vi "display_projector_one_color.vi"() -> ()   [LabVIEW 2019]
uses:
  <vilib>/vision/driver/IMAQdx.llb/IMAQdx Acquisition Mode.ctl
  ParametersGlobal.vi
  <vilib>/vision/NI_Vision_Development_Module.lvlib
  <vilib>/vision/driver/NI_Vision_Acquisition_Software.lvlib
panel:
  out "Processed Image":T1(plugin-control)
  out "Acquired Image 2":T1(plugin-control)
  out "Acquired Image":T1(plugin-control)
  in  "Single Color (T) Spatial Calibration Image (F)":bool=TRUE
  out "error out":errorcluster
  in  "Color Pixel Value":u32(colorbox)
  in  "Done":bool
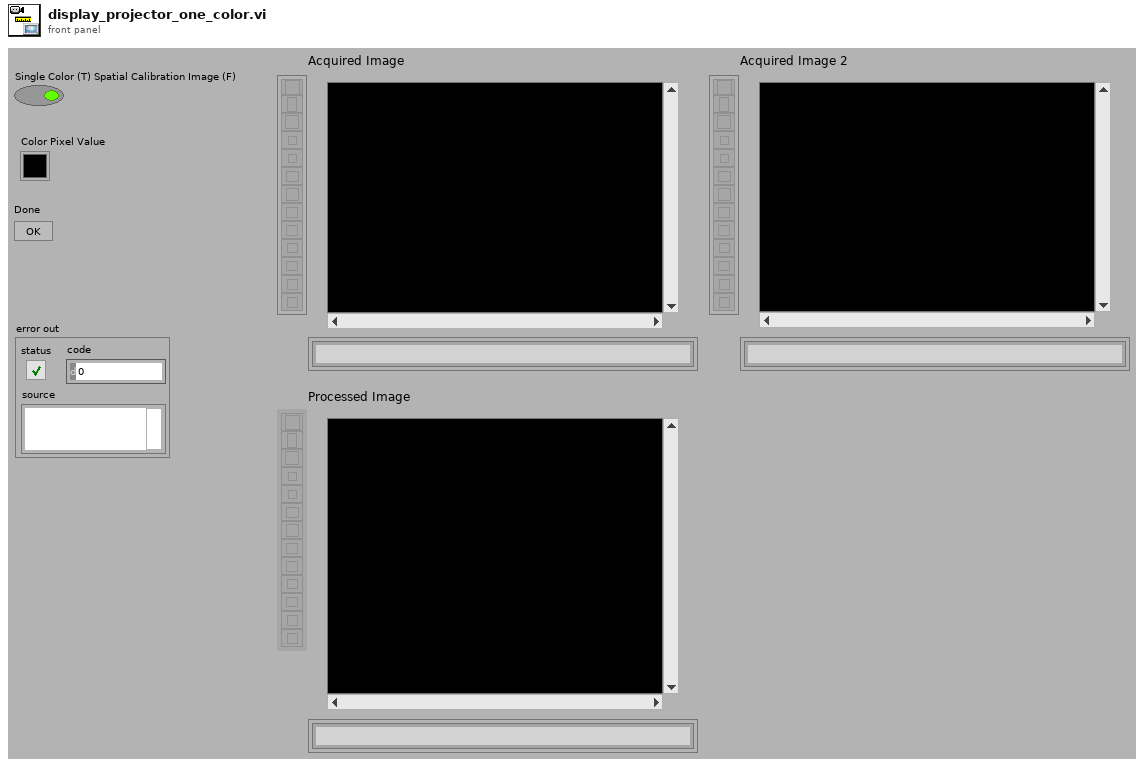
[diagram p1: front panel]
types:
  T1 = typedef "IMAQ Image.ctl" = refnum<image>
  T2 = typedef "NI_Vision_Acquisition_Software.lvlib/IMAQdx Acquisition Mode.ctl" = enum32{"One Shot", "Continuous"}
  T3 = typedef "Image Type" = u32
  T4 = typedef "IMAQdx.ctl" = refnum<k21>
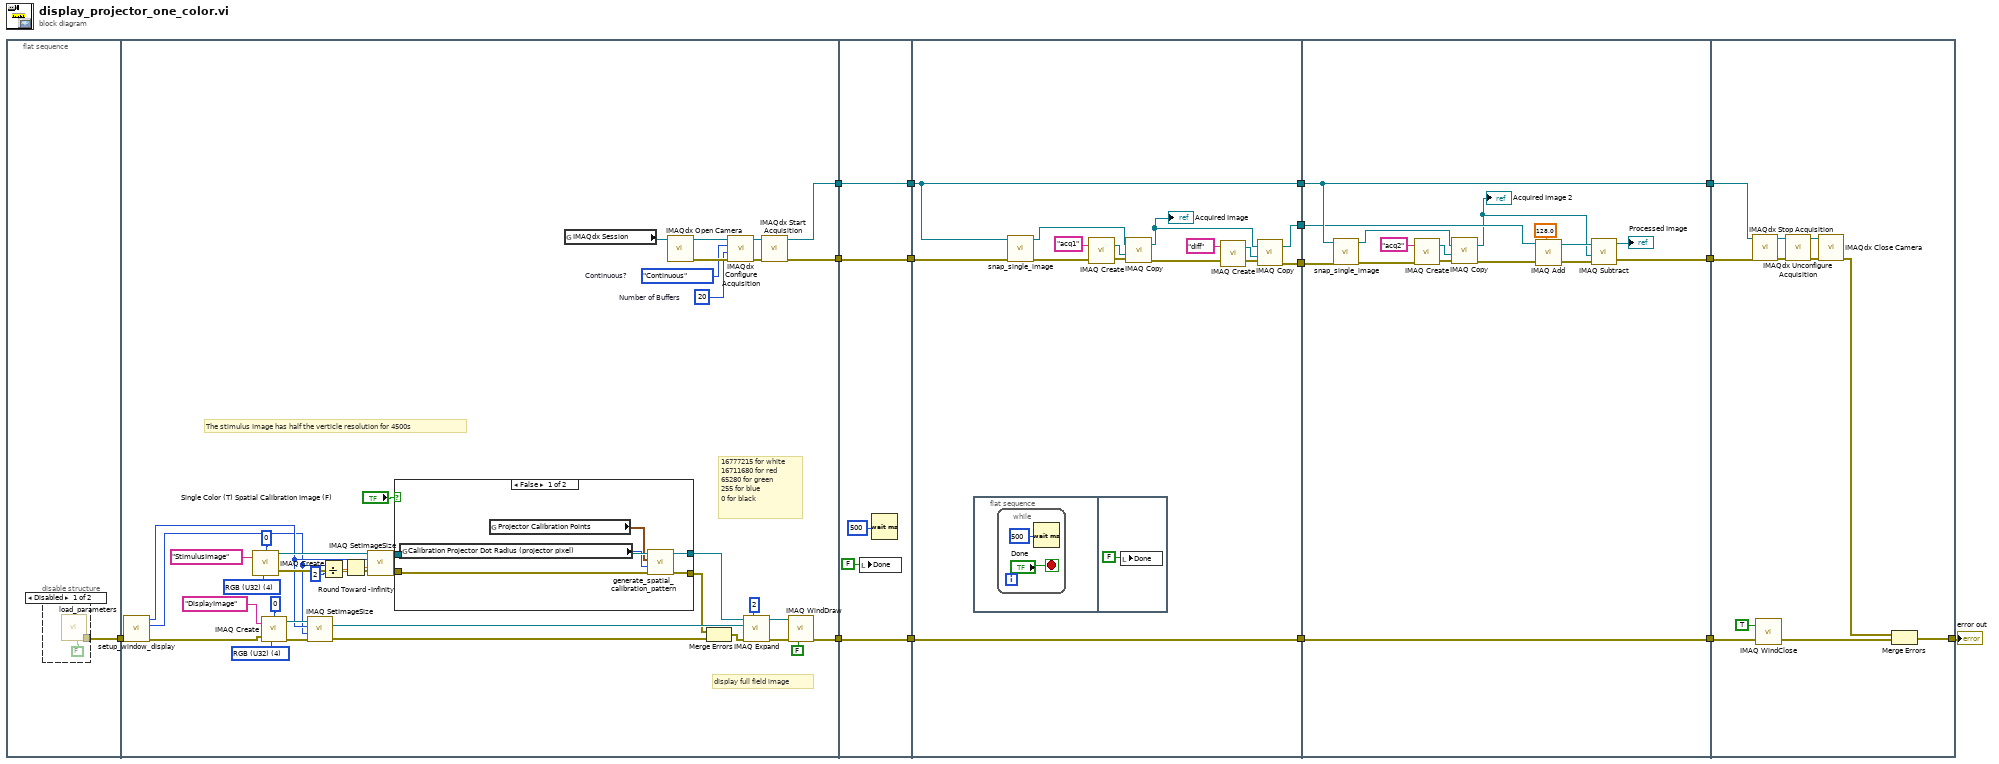
[diagram p0: block diagram]
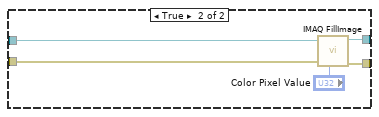
[diagram p3: hidden frame]
diagram:
  n1 = flat-sequence {
    tunnel: [w16] -> w14
    tunnel: [w51] -> w13
    tunnel: w14 -> [w33]
    tunnel: [w20] -> w11
    tunnel: [w19] -> w9
    tunnel: w13 -> [w73]
    tunnel: [w73] -> w12
    tunnel: w11 -> [w72]
    tunnel: [w72] -> w10
    tunnel: w9 -> [w71]
    tunnel: [w71] -> w8
    tunnel: [w88] -> w7
    tunnel: [w87] -> w4
    tunnel: w8 -> [w87]
    tunnel: w10 -> [w86]
    tunnel: w12 -> [w88]
    tunnel: [w75] -> w2
    tunnel: [w74] -> w1
    tunnel: w7 -> [w107]
    tunnel: [w107] -> w6
    tunnel: [w93] -> w5
    tunnel: w4 -> [w100]
    tunnel: [w100] -> w3
    tunnel: w2 -> [w101]
    tunnel: w1 -> [w99]
    tunnel: w6 -> [w118]
    tunnel: [w109] -> w15
    tunnel: w5 -> [w112]
    tunnel: w3 -> [w111]
    frame #0 {
      n2 = disable-structure shown="Disabled" {
        disable-tunnel: [w17 _] -> w16
        frame Disabled {
          n3 = call "load_parameters.vi"("Create Data Folder (T)"=FALSE) -> ("error out"=w17:errorcluster)  [unwired: 8 in, 2 out]
        }
        frame Enabled {
        }
      }
    }
    frame #1 {
      w23 = u32 20  # Number of Buffers
      w22 = IMAQdx_Acquisition_Mode."Continuous"  # Continuous?
      w48 = T3 4 items=["Grayscale (U8)", "Grayscale (I16)", "Grayscale (SGL)", "Complex (CSG)", "RGB (U32)", "HSL (U32)", "RGB (U64)"] ("Image Type")
      w53 = T3 4 items=["Grayscale (U8)", "Grayscale (I16)", "Grayscale (SGL)", "Complex (CSG)", "RGB (U32)", "HSL (U32)", "RGB (U64)"] ("Image Type")
      # "16777215 for white\n16711680 for red\n65280 for green\n255 for blue\n0 for black"
      # "The stimulus Image has half the verticle resolution for 4500s"
      # "display full field image"
      n4 = call "setup_window_display.vi"("error in (no error)"=w33) -> ("error out"=w34:errorcluster, "Height"=w35:i16, "Width"=w36:i16)  [unwired: 8 in]
      n5 = call "IMAQ Create"("Border Size"=0, "Image Name"="StimulusImage", "Image Type"=w48) -> ("New Image"=w47:T1, "error out"=w42:errorcluster)  [unwired: 2 in]
      n6 = call "IMAQ Create"("Border Size"=0, "Image Name"="DisplayImage", "Image Type"=w53, "error in (no error)"=w34) -> ("New Image"=w56:T1, "error out"=w57:errorcluster)  [unwired: 1 in]
      n7 = call "IMAQ SetImageSize"("error in (no error)"=w57, "Y Resolution"=w35, "X Resolution"=w36, "Image"=w56) -> ("error out"=w29:errorcluster, "Image Out"=w40:T1)  [unwired: 1 in]
      n8 = Divide(x=w35, y=2) -> (x/y=w44:dbl)
      n9 = Round Toward -Infinity(1:w44) -> (0:w45:dbl)
      n10 = call "IMAQ SetImageSize"("error in (no error)"=w42, "Y Resolution"=w45, "X Resolution"=w36, "Image"=w47) -> ("error out"=w41:errorcluster, "Image Out"=w46:T1)  [unwired: 1 in]
      n11 = case shown="False" "Single Color (T) Spatial Calibration Image (F)" {
        tunnel: w46 -> [w61 w68]
        tunnel: w41 -> [w63 w67]
        tunnel: [w60 w66] -> w37
        tunnel: [w62 w64] -> w30
        frame False {
          n12 = global read "ParametersGlobal.vi" "Calibration Projector Dot Radius (projector pixel)"() -> (w58:i32)
          n13 = global read "ParametersGlobal.vi" "Projector Calibration Points"() -> (w59:cluster{"X":dbl, "Y":dbl}[])
          n14 = call "generate_spatial_calibration_pattern.vi"("error in (no error)"=w63, "Dot Radius (Projector Pixels)"=w58, "Points Array"=w59, "StimulusImageIn"=w61) -> ("error out"=w62:errorcluster, "StimulusImageOut"=w60:T1)  [unwired: 6 in]
        }
        frame True {
          n15 = call "IMAQ FillImage"("Color Pixel Value"="Color Pixel Value", "error in (no error)"=w67, "Image"=w68) -> ("error out"=w64:errorcluster, "Image Out"=w66:T1)  [unwired: 7 in]
        }
      }
      n16 = global read "ParametersGlobal.vi" "IMAQdx Session"() -> (w21:T4)
      n17 = call <vilib>:"IMAQdx Open Camera.vi"("Session In"=w21) -> ("error out"=w26:errorcluster, "Session Out"=w27:T4)  [unwired: 9 in]
      n18 = Merge Errors(w30, w29) -> (w32:errorcluster)
      n19 = call <vilib>:"IMAQdx Configure Acquisition.vi"("error in"=w26, "Number of Buffers"=w23, "Continuous?"=w22, "Session In"=w27) -> ("error out"=w25:errorcluster, "Session Out"=w24:T4)  [unwired: 6 in]
      n20 = call "IMAQ Expand"("Y Duplication Step"=2, "error in (no error)"=w32, "Image Dst"=w40, "Image Src"=w37) -> ("error out"=w31:errorcluster, "Image Dst Out"=w39:T1)  [unwired: 6 in]
      n21 = call <vilib>:"IMAQdx Start Acquisition.vi"("error in"=w25, "Session In"=w24) -> ("error out"=w20:errorcluster, "Session Out"=w19:T4)  [unwired: 8 in]
      n22 = call "IMAQ WindDraw"("Resize to Image Size? (Y)"=FALSE, "error in (no error)"=w31, "Image"=w39) -> ("error out"=w51:errorcluster)  [unwired: 7 in, 1 out]
    }
    frame #2 {
      n23 = local write "Done"(FALSE) -> ()
      n24 = Wait (ms)(milliseconds to wait=500) -> ()  [unwired: 1 out]
    }
    frame #3 {
      n25 = flat-sequence {
        frame #0 {
          n26 = while {
            stop <- "Done" stop-if-true
            n27 = Wait (ms)(milliseconds to wait=500) -> ()  [unwired: 1 out]
          }
        }
        frame #1 {
          n28 = local write "Done"(FALSE) -> ()
        }
      }
      n29 = call "snap_single_image.vi"("error in (no error)"=w86, "Session In"=w87) -> ("error out"=w84:errorcluster, "Image Out"=w81:T1)  [unwired: 8 in]
      n30 = call "IMAQ Create"("Image Name"="acq1", "error in (no error)"=w84) -> ("New Image"=w82:T1, "error out"=w83:errorcluster)  [unwired: 3 in]
      n31 = call "IMAQ Copy"("error in (no error)"=w83, "Image Dst"=w82, "Image Src"=w81) -> ("error out"=w78:errorcluster, "Image Dst Out"=w76:T1)  [unwired: 3 in]
      "Acquired Image" <- w76
      n32 = call "IMAQ Create"("Image Name"="diff", "error in (no error)"=w78) -> ("New Image"=w79:T1, "error out"=w80:errorcluster)  [unwired: 3 in]
      n33 = call "IMAQ Copy"("error in (no error)"=w80, "Image Dst"=w79, "Image Src"=w76) -> ("error out"=w75:errorcluster, "Image Dst Out"=w74:T1)  [unwired: 3 in]
    }
    frame #4 {
      n34 = call "snap_single_image.vi"("error in (no error)"=w101, "Session In"=w100) -> ("error out"=w105:errorcluster, "Image Out"=w102:T1)  [unwired: 8 in]
      n35 = call "IMAQ Create"("Image Name"="acq2", "error in (no error)"=w105) -> ("New Image"=w103:T1, "error out"=w104:errorcluster)  [unwired: 3 in]
      n36 = call "IMAQ Copy"("error in (no error)"=w104, "Image Dst"=w103, "Image Src"=w102) -> ("error out"=w98:errorcluster, "Image Dst Out"=w94:T1)  [unwired: 3 in]
      "Acquired Image 2" <- w94
      n37 = call "IMAQ Add"("Image Src A"=w99, "Constant"=128.0, "error in (no error)"=w98) -> ("Image Dst Out"=w95:T1, "error out"=w96:errorcluster)  [unwired: 4 in]
      n38 = call "IMAQ Subtract"("Image Src A"=w95, "Image Src B"=w94, "error in (no error)"=w96) -> ("Image Dst Out"=→"Processed Image":T1, "error out"=w93:errorcluster)  [unwired: 4 in]
    }
    frame #5 {
      n39 = call <vilib>:"IMAQdx Stop Acquisition.vi"("error in"=w112, "Session In"=w111) -> ("error out"=w113:errorcluster, "Session Out"=w114:T4)  [unwired: 8 in]
      n40 = call "IMAQ WindClose"("Close All Windows (False)"=TRUE, "error in (no error)"=w118) -> ("error out"=w110:errorcluster)  [unwired: 4 in]
      n41 = call <vilib>:"IMAQdx Unconfigure Acquisition.vi"("error in"=w113, "Session In"=w114) -> ("error out"=w116:errorcluster, "Session Out"=w115:T4)  [unwired: 8 in]
      n42 = call <vilib>:"IMAQdx Close Camera.vi"("error in"=w116, "Session In"=w115) -> ("error out"=w108:errorcluster)  [unwired: 9 in]
      n43 = Merge Errors(w108, w110) -> (w109:errorcluster)
    }
  }
  "error out" <- w15
